vi "writeDBL.vi"(8 "error in (no error)":errorcluster, 10 "Input":dbl, 11 "ModbusBuffer in":refnum<class "ModbusBufferBuilder.lvclass">) -> (0 "error out":errorcluster, 3 "ModbusBuffer out":refnum<class "ModbusBufferBuilder.lvclass">)   [LabVIEW 2016, in "ModbusBufferBuilder.lvclass"]
uses:
  ModbusBufferBuilder.lvclass
  ModbusBufferBuilder.lvclass/ModbusBufferBuilder.ctl
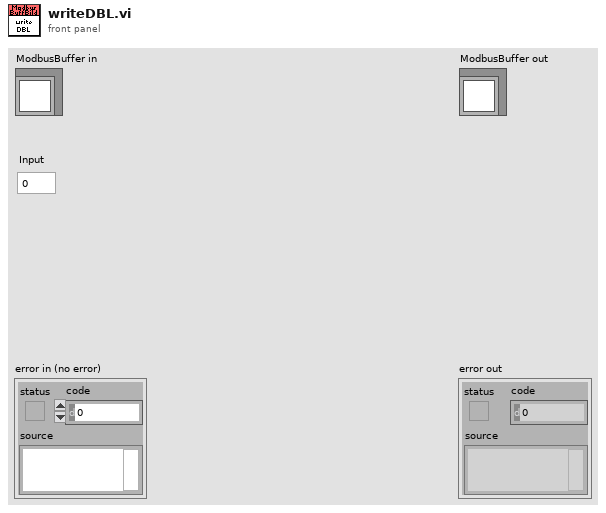
[diagram p1: front panel]
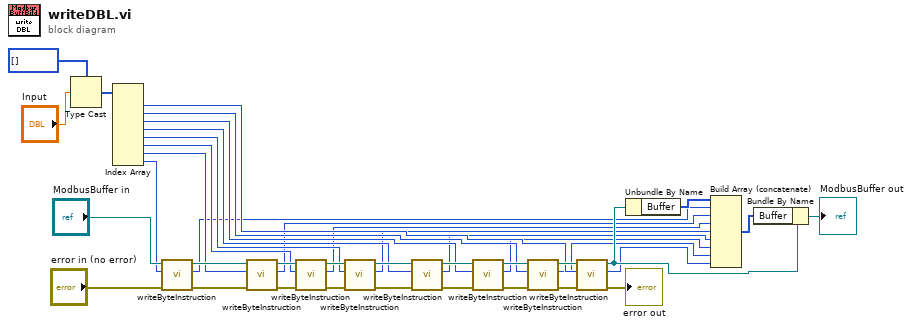
[diagram p0: block diagram]
diagram:
  n1 = Type Cast(type=u8[] [], x="Input") -> (*(type *) &x=w19:u8[])
  n2 = Index Array(array=w19) -> (element #1=w18:u8, element #2=w17:u8, element #3=w16:u8, element #4=w15:u8, element #5=w14:u8, element #6=w13:u8, element #7=w12:u8, element #8=w11:u8)  [unwired: 8 in]
  n3 = call "writeByteInstruction.vi"("error in (no error)"="error in (no error)", "Input"=w11, "ModbusBuffer in"="ModbusBuffer in") -> ("error out"=w29:errorcluster, "Output"=w9:u16, "ModbusBuffer out"=w38:refnum<class "ModbusBufferBuilder.lvclass">)  [unwired: 6 in]
  n4 = call "writeByteInstruction.vi"("error in (no error)"=w29, "Input"=w12, "ModbusBuffer in"=w38) -> ("error out"=w28:errorcluster, "Output"=w8:u16, "ModbusBuffer out"=w37:refnum<class "ModbusBufferBuilder.lvclass">)  [unwired: 6 in]
  n5 = call "writeByteInstruction.vi"("error in (no error)"=w28, "Input"=w13, "ModbusBuffer in"=w37) -> ("error out"=w27:errorcluster, "Output"=w7:u16, "ModbusBuffer out"=w36:refnum<class "ModbusBufferBuilder.lvclass">)  [unwired: 6 in]
  n6 = call "writeByteInstruction.vi"("error in (no error)"=w27, "Input"=w14, "ModbusBuffer in"=w36) -> ("error out"=w26:errorcluster, "Output"=w6:u16, "ModbusBuffer out"=w35:refnum<class "ModbusBufferBuilder.lvclass">)  [unwired: 6 in]
  n7 = call "writeByteInstruction.vi"("error in (no error)"=w26, "Input"=w15, "ModbusBuffer in"=w35) -> ("error out"=w25:errorcluster, "Output"=w5:u16, "ModbusBuffer out"=w34:refnum<class "ModbusBufferBuilder.lvclass">)  [unwired: 6 in]
  n8 = call "writeByteInstruction.vi"("error in (no error)"=w25, "Input"=w16, "ModbusBuffer in"=w34) -> ("error out"=w24:errorcluster, "Output"=w4:u16, "ModbusBuffer out"=w33:refnum<class "ModbusBufferBuilder.lvclass">)  [unwired: 6 in]
  n9 = call "writeByteInstruction.vi"("error in (no error)"=w24, "Input"=w17, "ModbusBuffer in"=w33) -> ("error out"=w23:errorcluster, "Output"=w3:u16, "ModbusBuffer out"=w32:refnum<class "ModbusBufferBuilder.lvclass">)  [unwired: 6 in]
  n10 = call "writeByteInstruction.vi"("error in (no error)"=w23, "Input"=w18, "ModbusBuffer in"=w32) -> ("error out"=→"error out":errorcluster, "Output"=w2:u16, "ModbusBuffer out"=w31:refnum<class "ModbusBufferBuilder.lvclass">)  [unwired: 6 in]
  n11 = Unbundle By Name(w31) -> ("Buffer"=w10:u16[])
  n12 = Build Array (concatenate)(w10, w9, w8, w7, w6, w5, w4, w3, w2) -> (w1:u16[])
  n13 = Bundle By Name(cluster=w31, "Buffer"=w1) -> (→"ModbusBuffer out":refnum<class "ModbusBufferBuilder.lvclass">)
